vi "LinearFilter_LowPassBW1.vi"(9 "SamplePeriod":dbl format="%13.5p", 11 "TimeConstant":dbl format="%13.5p") -> (3 "LINEAR_FILTER":T1 {"Outputs" format="%13.5g"; "Inputs" format="%13.5g"; "OutputGains" format="%13.5g"; "InputGains" format="%13.5g"})   [LabVIEW 2019, in "Trajectory_Library.lvlib"]
doc: "Creates a 1st order Butterworth low pass filter.\n\nMore information on this type of filter can be found at:\n\n https://en.wikipedia.org/wiki/Butterworth_filter\n\nInputs: \n - timeConstant - The discrete-time time constant in seconds.\n -samplePeriod - The period in seconds between samples taken by the user.\n\nOutputs:\n - LinearFilter - Created datat structure"
uses:
  Trajectory_Library.lvlib
  TypeDef/LINEAR_FILTER.ctl
  <vilib>/Rock Robotics/SystemInterfaces/NetworkCommunication/NetComm_UsageReport_report.vi
  Util_LibraryGlobals.vi
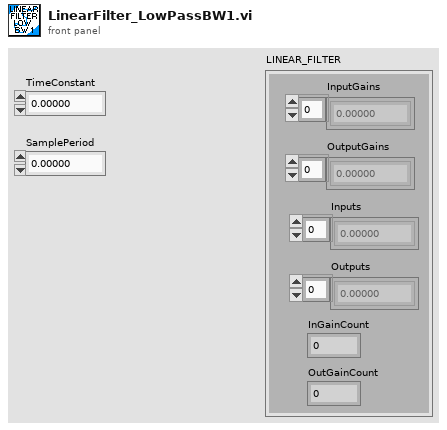
[diagram p1: front panel]
types:
  T1 = typedef "Trajectory_Library.lvlib/LINEAR_FILTER.ctl" = cluster{"InputGains":dbl[], "OutputGains":dbl[], "Inputs":dbl[], "Outputs":dbl[], "InGainCount":i32, "OutGainCount":i32}
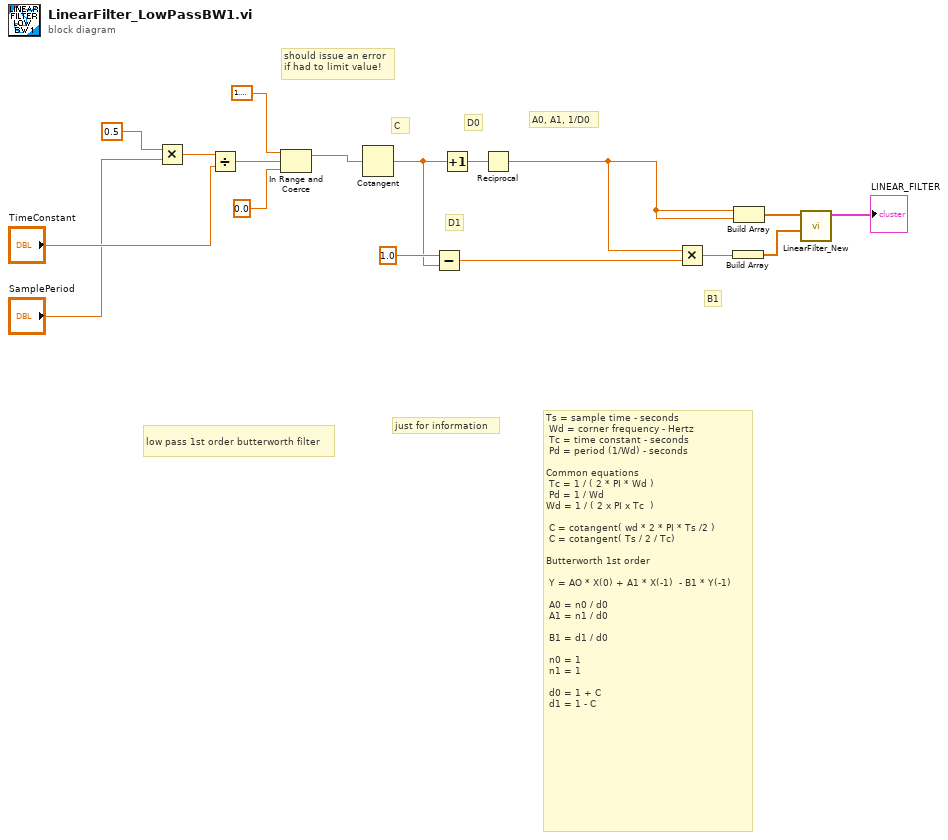
[diagram p0: block diagram]
diagram:
  # "A0, A1, 1/D0"
  # "B1"
  # "should issue an error\nif had to limit value!"
  # "Ts = sample time - seconds\n\tWd = corner frequency - Hertz\n\tTc = time constant - seconds\n\tPd = period (1/Wd) - seconds\n\nCommon equations\n\tTc = 1 / ( 2 * PI * Wd )\n\tPd = 1 / Wd\nWd = 1 / ( 2 x PI x Tc  )\n\t\n\tC = cotangent( wd * 2 * PI * Ts /2 )\n C = cotangent( Ts / 2 / Tc)\n\nButterworth 1st order\n\n\tY = AO * X(0) + A1 * X(-1)  - B1 * Y(-1) \n\n\tA0 = n0 / d0\n\tA1 = n1 / d0\n\n\tB1 = d1 / d0\n\n\tn0 = 1\n\tn1 = 1\n\n\td0 = 1 + C\n\td1 = 1 - C"
  # "D1"
  # "D0"
  # "C"
  # "just for information"
  # "low pass 1st order butterworth filter"
  n1 = Multiply(x=0.5, y="SamplePeriod") -> (x*y=w7:dbl)
  n2 = Divide(x=w7, y="TimeConstant") -> (x/y=w4:dbl)
  n3 = In Range and Coerce(upper limit=1.5707963267948966, x=w4, lower limit=0.0) -> (coerced(x)=w1:dbl)  [unwired: 1 out]
  n4 = Cotangent(1:w1) -> (0:w13:dbl)
  n5 = Subtract(x=1.0, y=w13) -> (x-y=w11:dbl)
  n6 = Increment(x=w13) -> (x+1=w12:dbl)
  n7 = Reciprocal(x=w12) -> (1/x=w9:dbl)
  n8 = Multiply(x=w9, y=w11) -> (x*y=w10:dbl)
  n9 = Build Array(w10) -> (w15:dbl[])
  n10 = Build Array(w9, w9) -> (w17:dbl[])
  n11 = call "LinearFilter_New.vi"("OutputGains"=w15, "InputGains"=w17) -> ("LINEAR_FILTER"=→"LINEAR_FILTER":T1)  [unwired: 9 in]
